vi "Power.vi"(11 "Power":dbl) -> ()   [LabVIEW 2014]
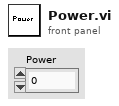
[diagram p1: front panel]
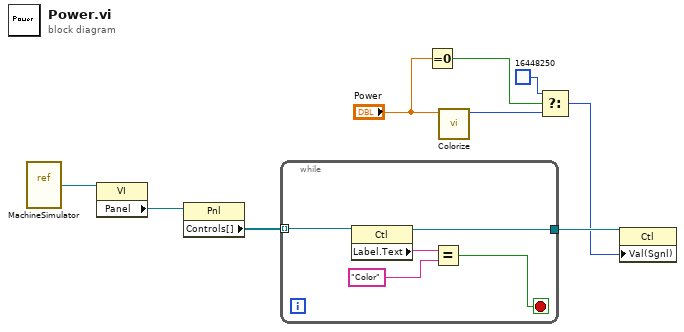
[diagram p0: block diagram]
diagram:
  n1 = vi-ref "MachineSimulator.vi"() -> (w6:refnum<vi>)
  n2 = property class="VI"(reference=w6) -> ("Panel"=w7:refnum<vi>)  [unwired: 1 in, 2 out]
  n3 = property class="Pnl"(reference=w7) -> ("Controls[]"=w9:refnum<vi>[])  [unwired: 1 in, 2 out]
  n4 = while {
    tunnel: w9 -> [w14] mode=indexing
    tunnel: [w10] -> w8
    stop <- w11 stop-if-true
    n5 = property class="Ctl"(reference=w14) -> (reference out=w10:refnum<vi>, "Label.Text"=w13:string)  [unwired: 1 in, 1 out]
    n6 = Equal?(x=w13, y="Color") -> (x = y?=w11:bool)
  }
  n7 = Equal To 0?(x="Power") -> (x = 0?=w3:bool)
  n8 = call "Colorize.vi"("ValueIn"="Power") -> ("ColorOut"=w1:u32)  [unwired: 10 in]
  n9 = Select(t=u32 16448250, s=w3, f=w1) -> (s? t:f=w4:u32)
  n10 = property class="Ctl"(reference=w8, "Val(Sgnl)"=w4) -> ()  [unwired: 1 in, 2 out]
